vi "onUnhandledDependencyError.vi"(7 "Stop on Unhandled Error (F)":bool, 8 "Unhandled Dependency Error":errorcluster, 9 "Dependency":refnum<class "SMO.lvclass">, 11 "SMO in":refnum<class "SMO.lvclass">) -> (0 "Unhandled error":errorcluster, 3 "SMO out":refnum<class "SMO.lvclass">)   [LabVIEW 2019, in "SMO.lvclass"]
doc: "JKI State Machine Objects (SMO) 1.3.0.56\nJKI - JKI\nCopyright (c) 2017, JKI"
uses:
  SMO.lvclass
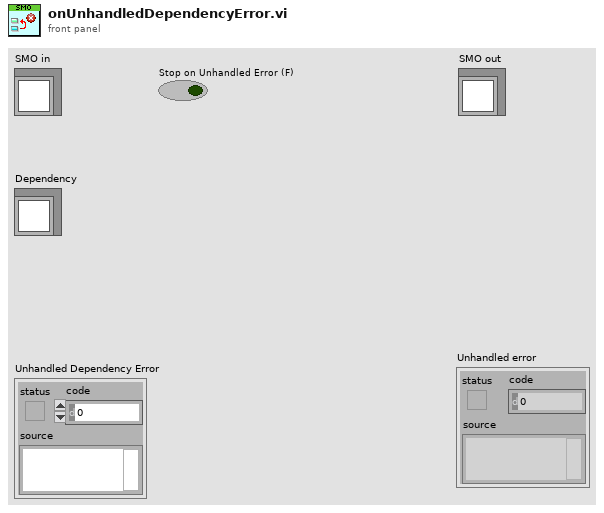
[diagram p1: front panel]
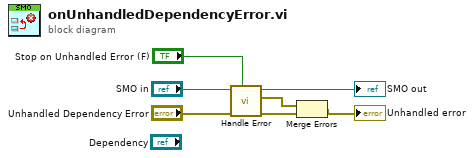
[diagram p0: block diagram]
diagram:
  n1 = call-dynamic "Handle Error.vi"("Stop on Unhandled Error (T)"="Stop on Unhandled Error (F)", "error in"="Unhandled Dependency Error", "SMO"="SMO in") -> ("handling error"=w3:errorcluster, "Unhandled error"=w2:errorcluster, "SMO out"=→"SMO out":refnum<class "SMO.lvclass">)  [unwired: 6 in]
  n2 = Merge Errors(w2, w3) -> (→"Unhandled error":errorcluster)
